vi "INI_SPI_Sysl.vi"(3 "MCListbox Ref":refnum<vi>, 9 "MListBox Row":u16=2 max=8, 10 "config":T1={"ClockRate"=50000, "LatencyTimer"=255, "configOptions 24-31"=0, "configOptions 16-23"=0, "configOptions 8-15"=0, "configOptions 0-7"=32, "Pin"=0, "reserved"=0} {"configOptions 24-31" format="%x"; "configOptions 16-23" format="%x"; "configOptions 8-15" format="%x"; "configOptions 0-7" format="%x"}, 11 "Device INI Config File Path":path=path "D:/LABVIEW/Examples/INI Devices/DeviceConfig.ini") -> (0 "error out":errorcluster, 1 "Dev OK":bool, 2 "Handle":u32)   [LabVIEW 2018]
uses:
  <vilib>/Utility/miscctls.llb/LVRowAndColumnTypeDef.ctl
  <vilib>/Utility/config.llb/Read Key (String).vi
  <vilib>/Utility/config.llb/Read Key (U32).vi
  <vilib>/Utility/config.llb/NI_LVConfig.lvlib
panel:
  # "configOptions\nThis member provides a way to enable/disable features\n\tspecific to the protocol that are implemented in the chip\n\tBIT1-0=CPOL-CPHA:\t00 - MODE0 - data captured on rising edge, propagated on falling\n \t\t\t\t\t\t01 - MODE1 - data captured on falling edge, propagated on rising\n \t\t\t\t\t\t10 - MODE2 - data captured on falling edge, propagated on rising\n \t\t\t\t\t\t11 - MODE3 - data captured on rising edge, propagated on falling\n\tBIT4-BIT2: 000 - A/B/C/D_DBUS3=ChipSelect\n\t\t\t : 001 - A/B/C/D_DBUS4=ChipSelect\n \t\t\t : 010 - A/B/C/D_DBUS5=ChipSelect\n \t\t\t : 011 - A/B/C/D_DBUS6=ChipSelect\n \t\t\t : 100 - A/B/C/D_DBUS7=ChipSelect\n \tBIT5: ChipSelect is active high if this bit is 0\n\tBIT6 -BIT31\t\t: Reserved"
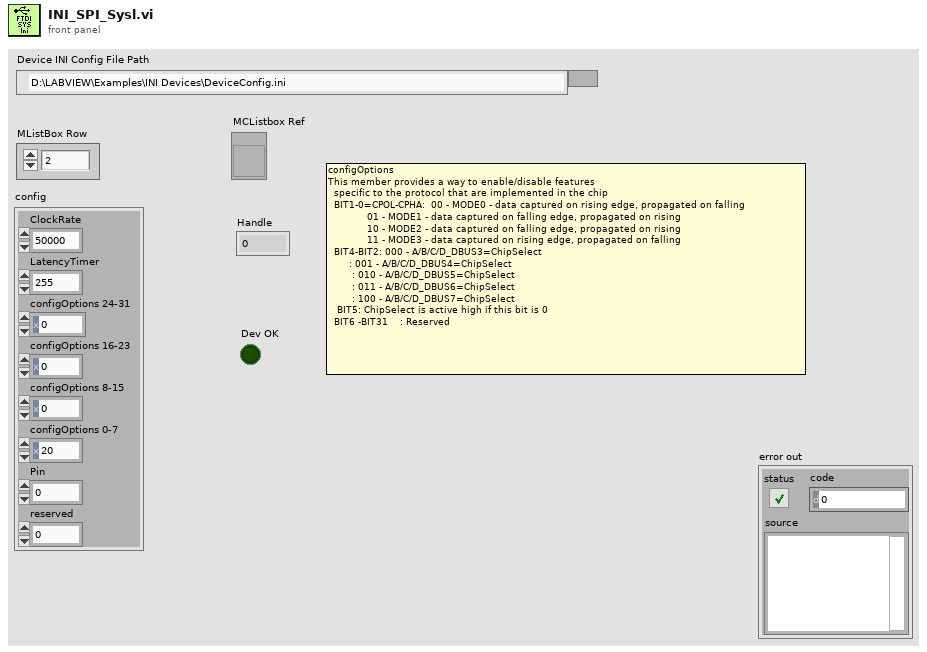
[diagram p1: front panel]
types:
  T1 = cluster{"ClockRate":u32, "LatencyTimer":u8, "configOptions 24-31":i8, "configOptions 16-23":i8, "configOptions 8-15":i8, "configOptions 0-7":u32, "Pin":u32, "reserved":u16}
  T2 = typedef "LVRowAndColumnTypeDef.ctl" = cluster{"Row":i32, "Column":i32}
  T3 = typedef "NI_LVConfig.lvlib/Config Data RefNum.ctl" = refnum<k1>
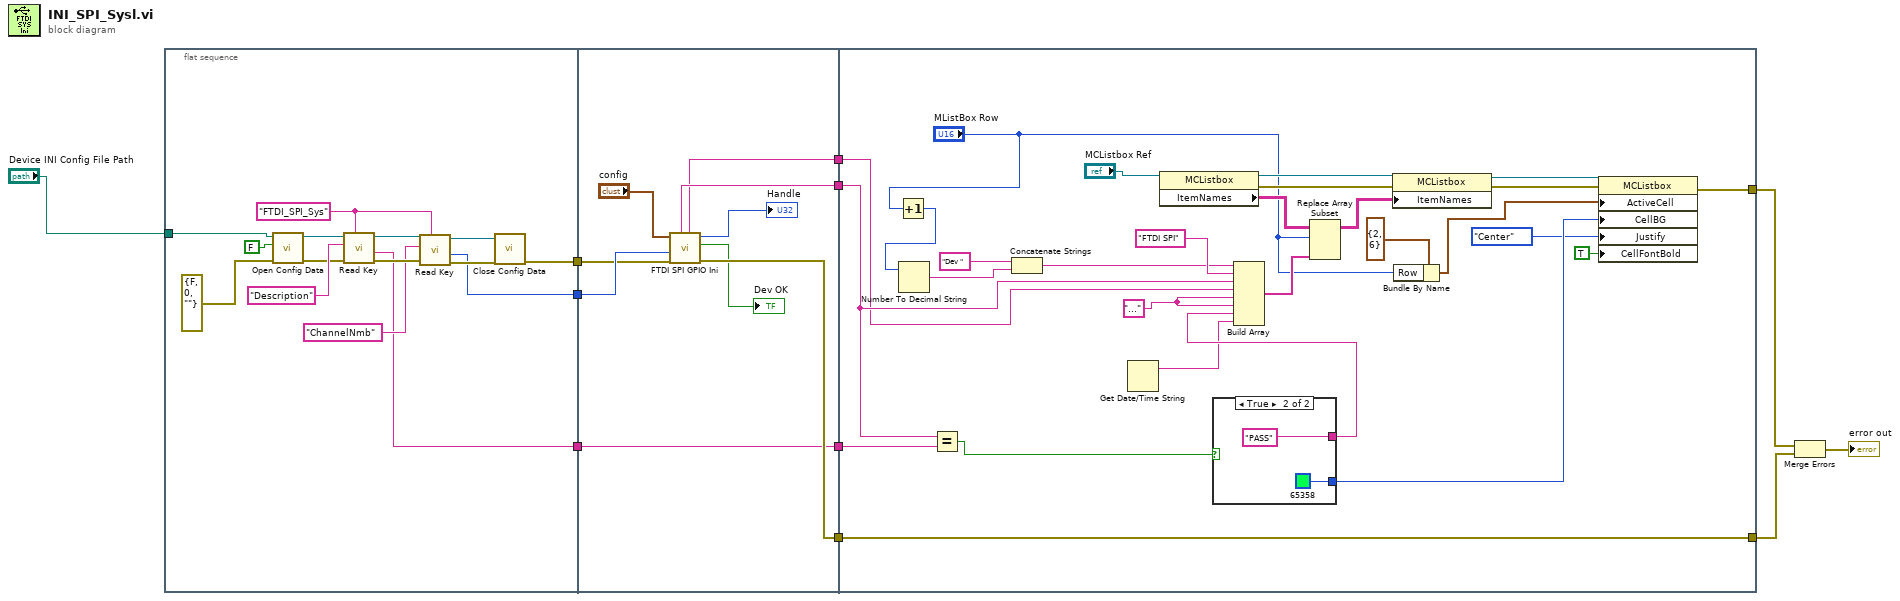
[diagram p0: block diagram]
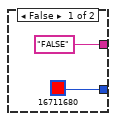
[diagram p2: hidden frame]
diagram:
  n1 = flat-sequence {
    tunnel: "Device INI Config File Path" -> [w21]
    tunnel: [w14] -> w11
    tunnel: [w13] -> w10
    tunnel: [w12] -> w3
    tunnel: w11 -> [w34]
    tunnel: w10 -> [w33]
    tunnel: [w31] -> w5
    tunnel: [w30] -> w4
    tunnel: w3 -> [w30]
    tunnel: [w29] -> w2
    tunnel: [w28] -> w1
    tunnel: [w43] -> w7
    tunnel: [w42] -> w6
    tunnel: w5 -> [w42]
    tunnel: w4 -> [w41]
    tunnel: w2 -> [w39]
    tunnel: w1 -> [w38]
    frame #0 {
      w18 = "FTDI_SPI_Sys" ("section")
      n2 = call <vilib>:"Open Config Data.vi"("error in (no error)"=errorcluster {"status"=FALSE, "code"=0, "source"=""} ("error constant"), "create file if necessary (T)"=FALSE, "configuration file path"=w21) -> ("error out"=w24:errorcluster, "refnum"=w23:T3)  [unwired: 6 in, 1 out]
      n3 = call-poly <vilib>:"Read Key.vi"("section"=w18, "error in (no error)"=w24, "key"="Description", "refnum"=w23) -> ("error out"=w17:errorcluster, "value"=w12:string, "refnum out"=w20:T3)  [unwired: 4 in, 1 out]
      n4 = call-poly <vilib>:"Read Key.vi"("section"=w18, "error in (no error)"=w17, "key"="ChannelNmb", "refnum"=w20) -> ("error out"=w16:errorcluster, "value"=w14:u32, "refnum out"=w19:T3)  [unwired: 4 in, 1 out]
      n5 = call <vilib>:"Close Config Data.vi"("error in (no error)"=w16, "refnum"=w19) -> ("error out"=w13:errorcluster)  [unwired: 8 in, 1 out]
    }
    frame #1 {
      n6 = call "FTDI SPI GPIO Ini.vi"("error in (no error)"=w33, "Channel Nmb"=w34, "config"="config") -> ("error out"=w31:errorcluster, "Ini Status"=→"Dev OK":bool, "handle out"=→"Handle":u32, "Serial number"=w28:string, "Description"=w29:string)  [unwired: 4 in]
    }
    frame #2 {
      w63 = "..."
      n7 = Increment(x="MListBox Row") -> (x+1=w37:u16)
      n8 = Number To Decimal String(number=w37) -> (decimal integer string=w60:string)  [unwired: 1 in]
      n9 = Equal?(x=w39, y=w41) -> (x = y?=w40:bool)
      n10 = Concatenate Strings("Dev ", w60) -> (w61:string)
      n11 = Get Date/Time String() -> (date string=w53:string)  [unwired: 3 in, 1 out]
      n12 = property class="MCListbox"(reference="MCListbox Ref") -> (reference out=w51:refnum<vi>, error out=w50:errorcluster, "ItemNames"=w49:string[][])  [unwired: 1 in]
      n13 = case shown="True" w40 {
        tunnel: [u32 16711680 u32 65358] -> w56
        tunnel: ["FALSE" ("element") "PASS" ("element")] -> w57
        frame False {
        }
        frame True {
        }
      }
      n14 = Build Array(w61, "FTDI SPI", w39, w38, w63, w63, w57, w53) -> (w47:string[])
      n15 = Replace Array Subset(array=w49, new element=w47, index (row)="MListBox Row") -> (w48:string[][])  [unwired: 1 in]
      n16 = property class="MCListbox"(reference=w51, error in=w50, "ItemNames"=w48) -> (reference out=w46:refnum<vi>, error out=w45:errorcluster)
      n17 = Bundle By Name(cluster=T2 {"Row"=2, "Column"=6} ("Active Cell:Active Cell"), "Row"="MListBox Row") -> (w55:T2)
      n18 = property class="MCListbox"(reference=w46, error in=w45, "ActiveCell"=w55, "CellBG"=w56, "Justify"=enum16{"Left", "Center", "Right"}."Center" ("Active Cell:Cell Justification"), "CellFontBold"=TRUE ("Active Cell:Cell Font:Bold")) -> (error out=w43:errorcluster)  [unwired: 1 out]
    }
  }
  n19 = Merge Errors(w7, w6) -> (→"error out":errorcluster)
